vi "Convert Complex Cluster to Phase.vi"(0 "IQ data (complex) In":cluster{"t0":dbl, "dt":dbl, "Y":cdb[]}={"t0"=0.0, "dt"=1.0, "Y"=[]} {"Y" format="%.2f"; "dt" format="%.2f"; "t0" format="%.2f"}, 7 "phase unit":i32(ring) items=["radian in, radian out", "radian in, degree out", "degree in, degree out", "degree in, radian out"], 11 "Error In":errorcluster) -> (4 "Phase Out":cluster{"t0":dbl, "dt":dbl, "Y":dbl[]}={"t0"=0.0, "dt"=1.0, "Y"=[]} {"Y" min=0.0 max=127.0 format="%.6f"; "dt" format="%.2f"; "t0" format="%.2f"}, 15 "Error Out":errorcluster)   [LabVIEW 2019]
uses:
  <vilib>/Analysis/NI_AALPro.lvlib
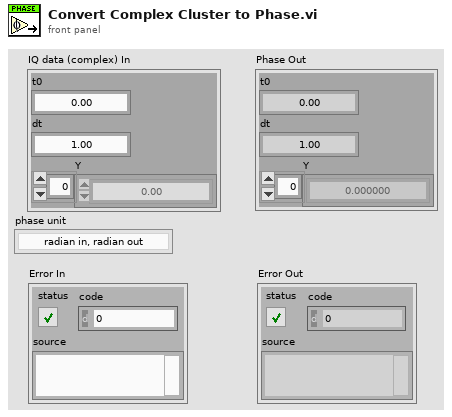
[diagram p1: front panel]
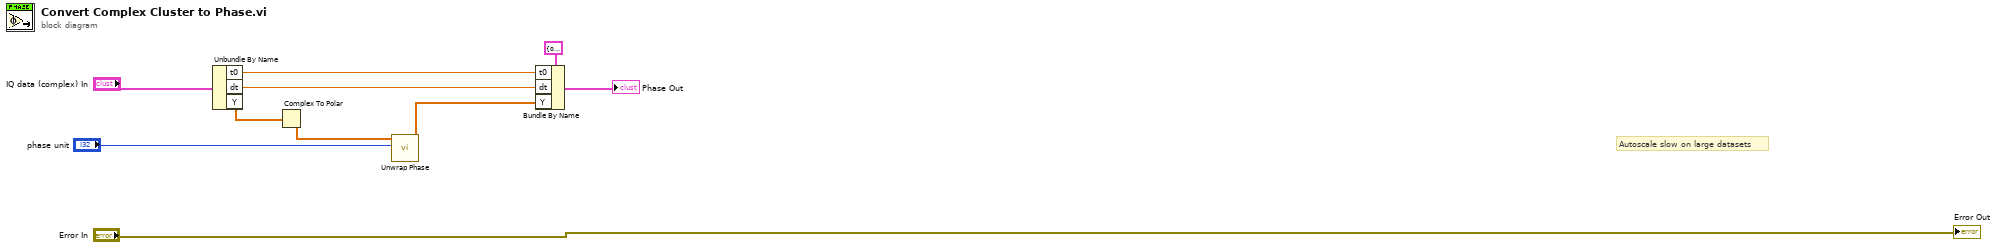
[diagram p0: block diagram]
diagram:
  # "Autoscale slow on large datasets"
  n1 = Unbundle By Name("IQ data (complex) In") -> ("t0"=w8:dbl, "dt"=w7:dbl, "Y"=w3:cdb[])
  n2 = Complex To Polar(r * e^(i*theta)=w3) -> (theta=w2:dbl[])  [unwired: 1 out]
  n3 = call <vilib>:"Unwrap Phase.vi"("phase unit"="phase unit", "Phase"=w2) -> ("Unwrapped Phase"=w1:dbl[])  [unwired: 8 in, 1 out]
  n4 = Bundle By Name(cluster=cluster{"t0":dbl, "dt":dbl, "Y":dbl[]} {"t0"=0.0, "dt"=1.0, "Y"=[]} ("Magnitude Out"), "t0"=w8, "dt"=w7, "Y"=w1) -> (→"Phase Out":cluster{"t0":dbl, "dt":dbl, "Y":dbl[]})
  "Error Out" <- "Error In"
